vi "Choreo_Util_AllianceFlipY.vi"(11 "Y":dbl) -> (3 "FlippedY":dbl)   [LabVIEW 2019, in "ChoreoLib.lvlib"]
doc: "Flips the Y coordinate.\n \nInputs: \n -- y - double - The Y coordinate to flip.\n\nOutputs:\n -- FlippedY - double - The flipped Y coordinate."
uses:
  ChoreoLib.lvlib
  Choreo_Choreo_Globals.vi
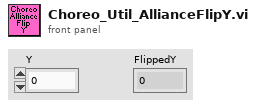
[diagram p1: front panel]
types:
  T1 = typedef "ChoreoLib.lvlib/Choreo_Util_AllianceFlipType.ctl" = enum16{"MIRRORED", "ROTATE_AROUND"}
  T2 = cluster{"Year":i32, "AllianceFlipType":T1, "FieldLength":dbl, "FieldWidth":dbl}
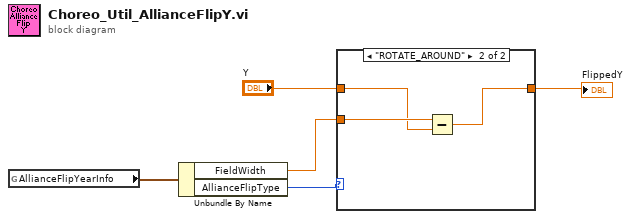
[diagram p0: block diagram]
diagram:
  n1 = global read "Choreo_Choreo_Globals.vi" "AllianceFlipYearInfo"() -> (w5:T2)
  n2 = Unbundle By Name(w5) -> ("FieldWidth"=w1:dbl, "AllianceFlipType"=w4:T1)
  n3 = case shown="\"ROTATE_AROUND\"" w4 {
    tunnel: "Y" -> [w6 w8]
    tunnel: [w6 w7] -> w2
    tunnel: w1 -> [_ w9]
    frame "MIRRORED" {
    }
    frame "ROTATE_AROUND" {
      n4 = Subtract(x=w9, y=w8) -> (x-y=w7:dbl)
    }
  }
  "FlippedY" <- w2
